vi "Calculate_Cost_F()-4.vi"(0 "[IN] Subtracks":T2(array[cluster]), 1 "[IN] Still connected\ntracks in group":T1, 2 "[IN] Max angle":dbl, 3 "[IN] Areas particles\nPrimary Detected":dbl[][](array[numeric]), 7 "[IN] Index of Earliest \nProblem Point Inside":i32, 9 "[IN] # of Longest track\nInside the Tracks Group":i32, 11 "error IN":errorcluster, 12 "[IN] Primary \n(X,Y) Detected":dbl[][](array[numeric]), 13 "[IN] Potentially\nMoving (X,Y)":dbl[][](array[numeric]), 14 "[IN] Dot matrix with statuses \nfor potentially moving dots":i16[][](array[numeric])) -> (4 "[OUT] Cost function":i8[](array[numeric]), 15 "error OUT":errorcluster)   [LabVIEW 2013]
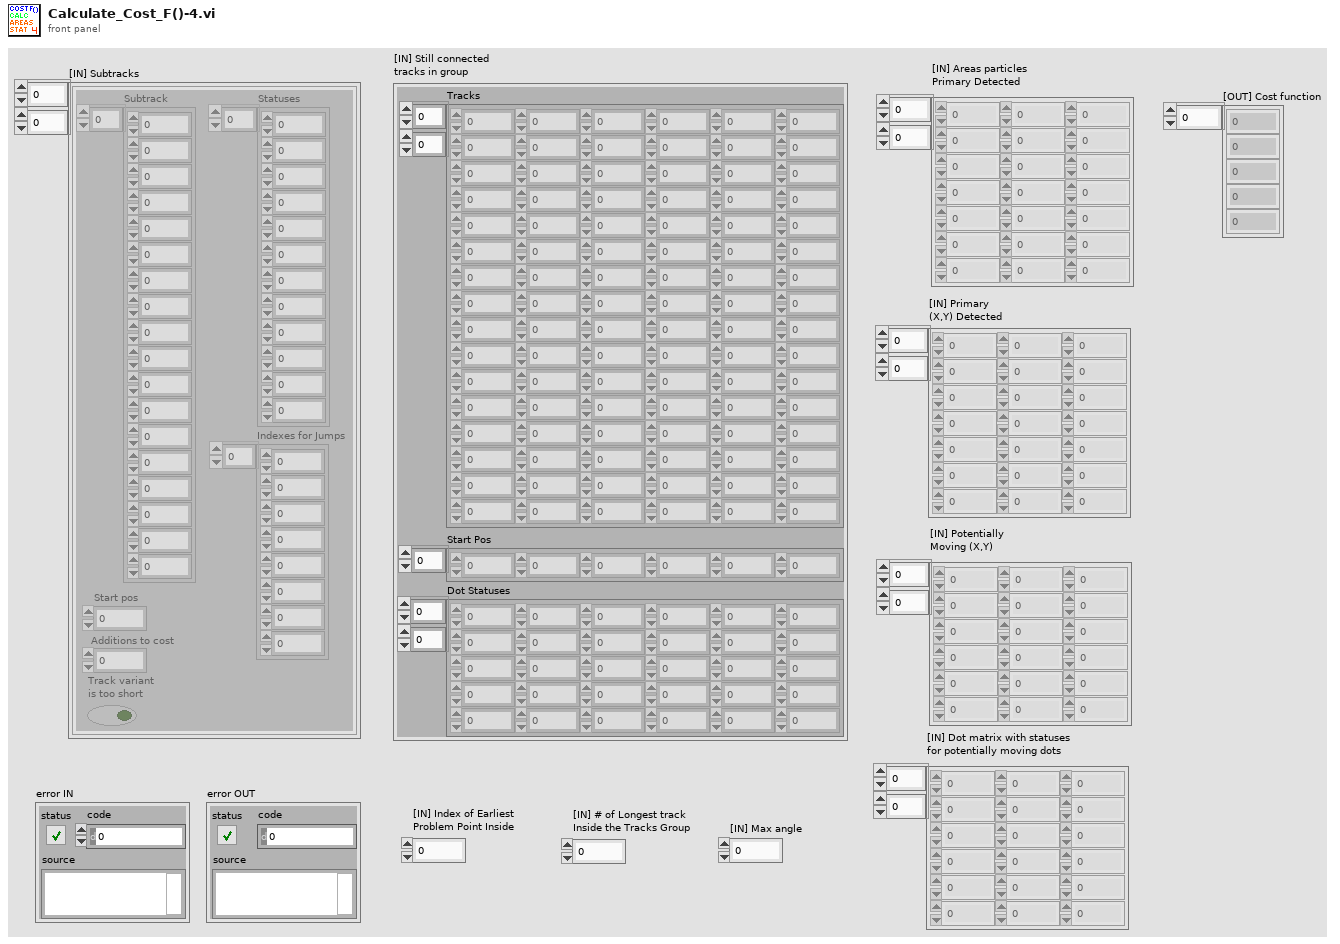
[diagram p1: front panel]
types:
  T1 = cluster{"Tracks":dbl[][], "Start Pos":i32[], "Dot Statuses":i16[][]}
  T2 = cluster{"Subtrack":dbl[], "Statuses":i16[], "Start pos":i32, "Additions to cost":i32, "Track variant \nis too short":bool, "Indexes for Jumps":i32[]}[][]
  T3 = cluster{"Subtrack":dbl[], "Statuses":i16[], "Start pos":i32, "Additions to cost":i32, "Track variant \nis too short":bool, "Indexes for Jumps":i32[]}[]
  T4 = cluster{"Subtrack":dbl[], "Statuses":i16[], "Start pos":i32, "Additions to cost":i32, "Track variant \nis too short":bool, "Indexes for Jumps":i32[]}
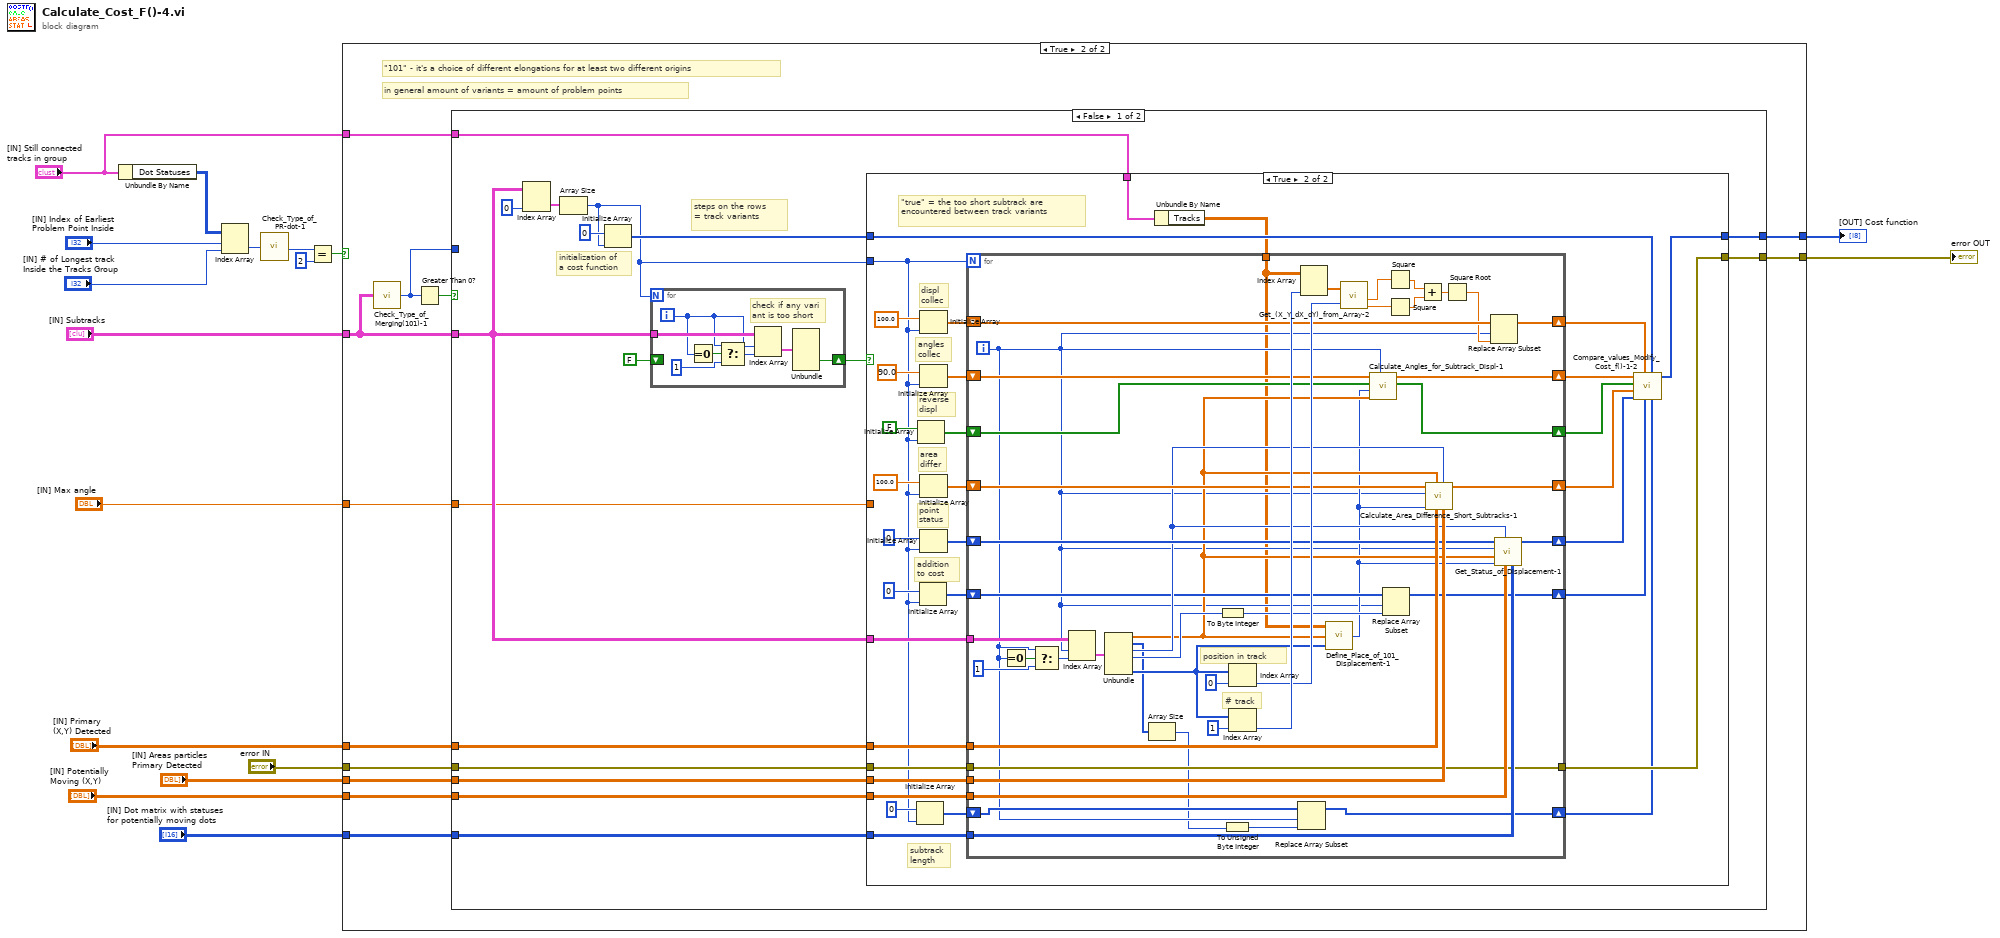
[diagram p0: block diagram]
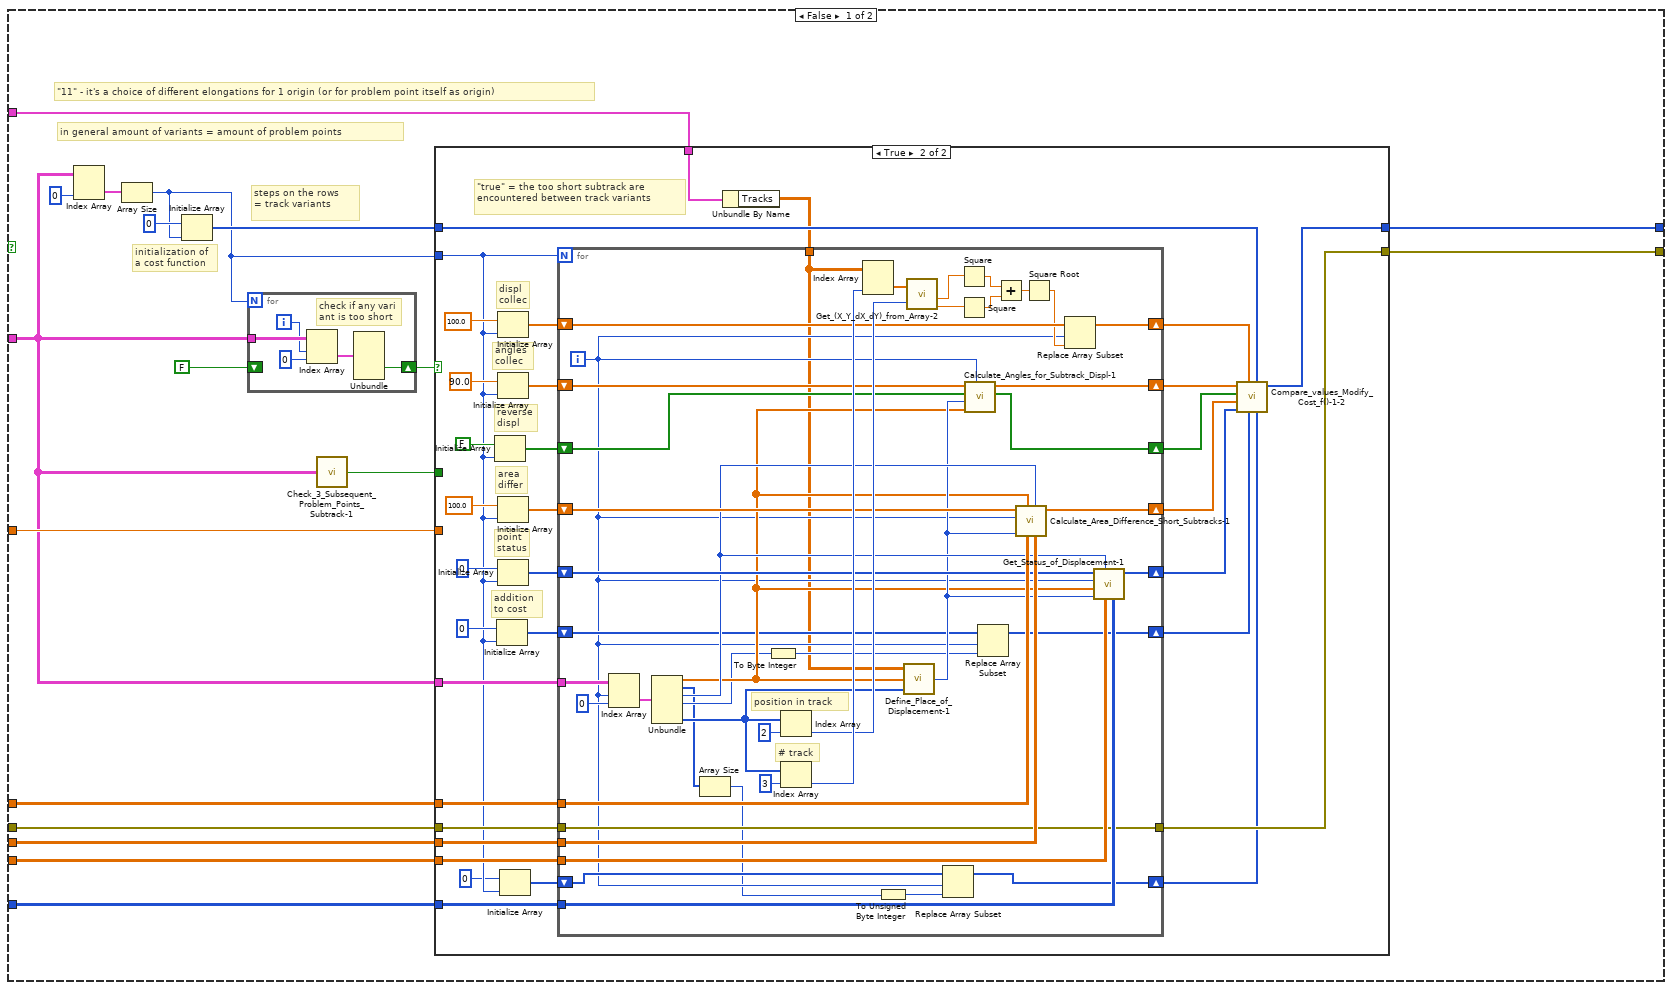
[diagram p2: hidden frame]
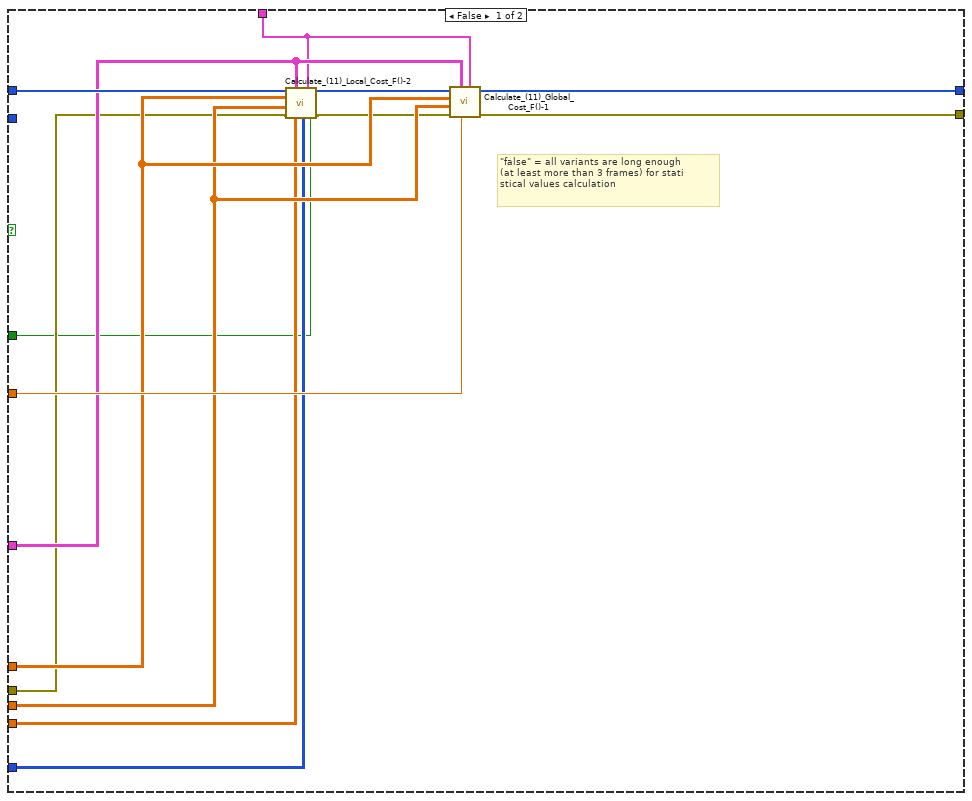
[diagram p3: hidden frame]
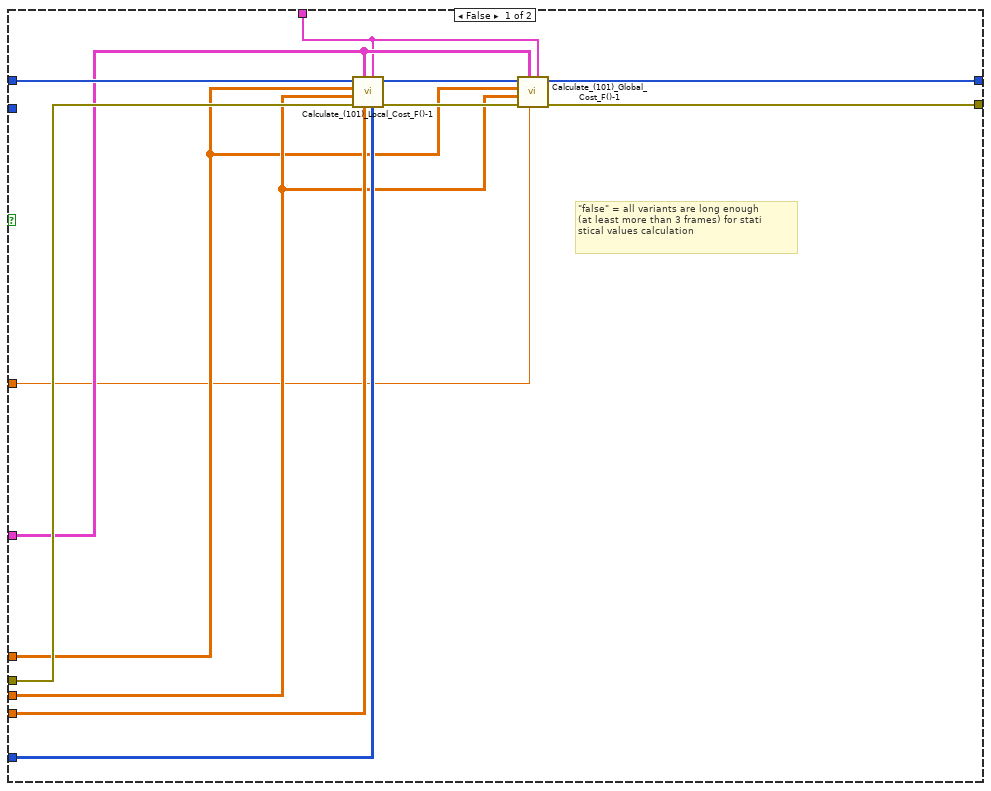
[diagram p4: hidden frame]
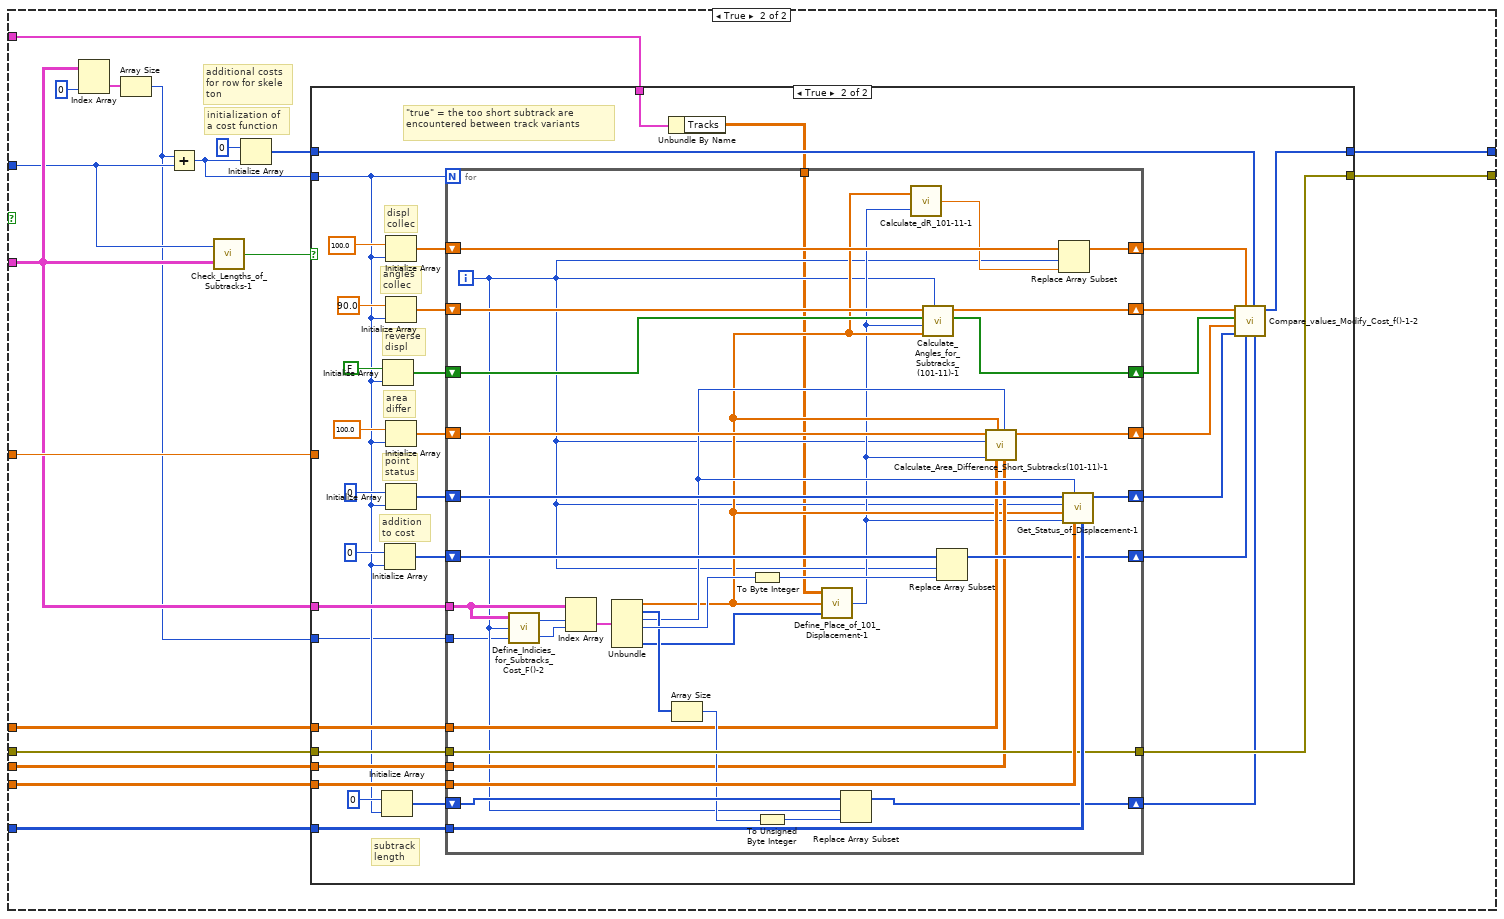
[diagram p5: hidden frame]
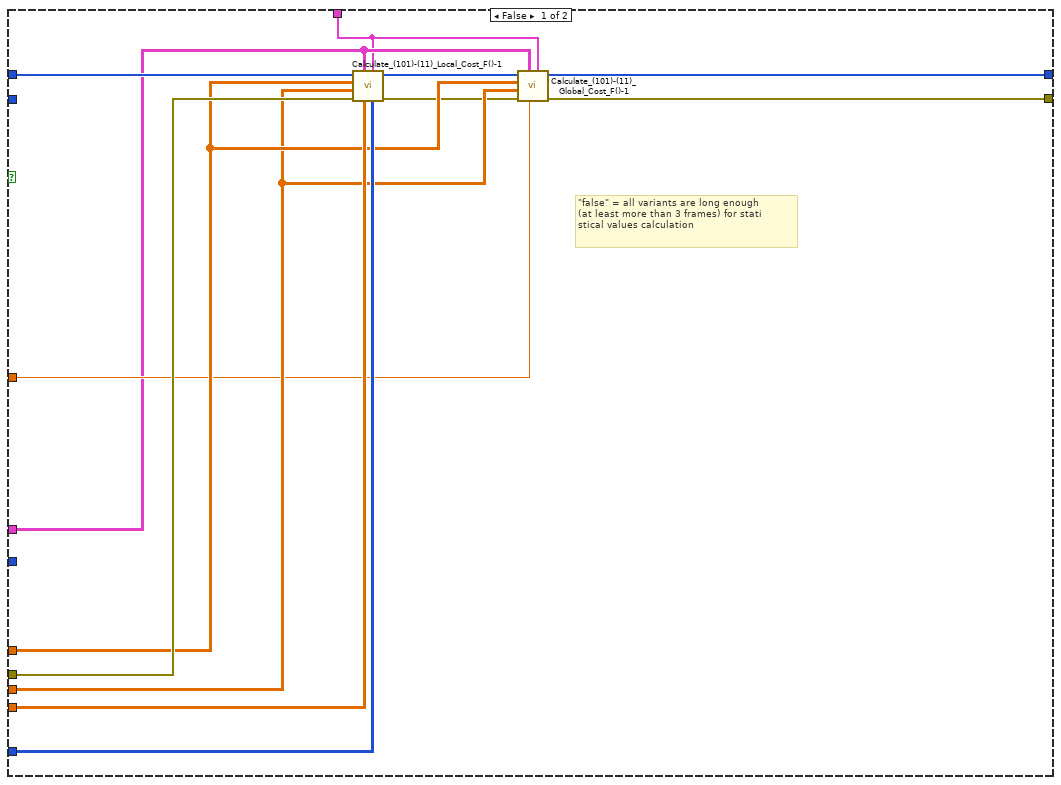
[diagram p6: hidden frame]
diagram:
  n1 = Unbundle By Name("[IN] Still connected\ntracks in group") -> ("Dot Statuses"=w15:i16[][])
  n2 = Index Array(array=w15, index (row)="[IN] Index of Earliest \nProblem Point Inside", index (col)="[IN] # of Longest track\nInside the Tracks Group") -> (element=w14:i16)
  n3 = call "Check_Type_of_PR-dot-1.vi"("[IN] dot status"=w14) -> ("[OUT] Type of\nproblem dot"=w17:i32)
  n4 = Equal?(x=w17, y=2) -> (x = y?=w13:bool)
  n5 = case shown="True" w13 {
    tunnel: "[IN] Subtracks" -> [w19 w135]
    tunnel: "[IN] Still connected\ntracks in group" -> [w29 w132]
    tunnel: "[IN] Primary \n(X,Y) Detected" -> [w28 w142]
    tunnel: "[IN] Areas particles\nPrimary Detected" -> [w27 w140]
    tunnel: "[IN] Potentially\nMoving (X,Y)" -> [w26 w139]
    tunnel: "[IN] Dot matrix with statuses \nfor potentially moving dots" -> [w25 w138]
    tunnel: "error IN" -> [w24 w141]
    tunnel: "[IN] Max angle" -> [w23 w143]
    tunnel: [w22 w137] -> w2
    tunnel: [w21 w136] -> w1
    frame False {
      # "initialization of \na cost function"
      # "steps on the rows\n= track variants"
      # "in general amount of variants = amount of problem points"
      # "\"11\" - it's a choice of different elongations for 1 origin (or for problem point itself as origin)"
      n6 = Index Array(array=w19, index (col)=0 ("disabled index (col)")) -> (element=w34:T3)  [unwired: 1 in]
      n7 = Array Size(array=w34) -> (size(s)=w20:i32)
      n8 = Initialize Array(i8 0, w20) -> (w30:i8[])
      n9 = for {
        N: w20 -> [_]
        tunnel: w19 -> [w131]
        shift-right: [w127] -> w31
        shift-left: FALSE -> [_]
        i -> [w128]
        # "check if any vari\nant is too short"
        n10 = Index Array(array=w131, index (row)=w128, index (col)=0 ("disabled index (col)")) -> (element=w129:T4)
        n11 = Unbundle(w129) -> ("Track variant \nis too short"=w127:bool)  [unwired: 5 out]
      }
      n12 = call "Check_3_Subsequent_Problem_Points_Subtrack-1.vi"("[IN] Subtracks"=w19) -> ("[OUT] 3 Subsequent problem points in subtrack"=w18:bool)
      n13 = case shown="True" w31 {
        tunnel: w30 -> [w46 w58]
        tunnel: w20 -> [_ w63]
        tunnel: w19 -> [w45 w82]
        tunnel: w29 -> [w44 w51]
        tunnel: w28 -> [w43 w73]
        tunnel: w27 -> [w42 w72]
        tunnel: w26 -> [w40 w69]
        tunnel: w25 -> [w39 w68]
        tunnel: w24 -> [w41 w65]
        tunnel: w23 -> [w49 _]
        tunnel: [w48 w57] -> w22
        tunnel: [w47 w64] -> w21
        tunnel: w18 -> [w36 _]
        frame False {
          # "\"false\" = all variants are long enough\n(at least more than 3 frames) for stati\nstical values calculation"
          n14 = call "Calculate_(11)_Local_Cost_F()-2.vi"("[IN] Cost function"=w46, "[IN] Subtracks"=w45, "[IN] Still connected\ntracks in group"=w44, "[IN] Primary \n(X,Y) Detected"=w43, "[IN] Areas particles\nPrimary Detected"=w42, "error IN"=w41, "[IN] Potentially\nMoving (X,Y)"=w40, "[IN] Dot matrix with statuses \nfor potentially moving dots"=w39, "[IN] 3 Subsequent problem points in subtrack"=w36) -> ("[OUT] Cost function"=w37:i8[], "error OUT"=w38:errorcluster)  [unwired: 5 in]
          n15 = call "Calculate_(11)_Global_Cost_F()-1.vi"("[IN] Still connect\ned tracks in group"=w44, "[IN] Max angle"=w49, "[IN] Subtracks"=w45, "error IN"=w38, "[IN] Areas particles\nPrimary Detected"=w42, "[IN] Primary \n(X,Y) Detected"=w43, "[IN] Cost function"=w37) -> ("error OUT"=w47:errorcluster, "[OUT] Cost function"=w48:i8[])  [unwired: 3 in]
        }
        frame True {
          # "addition \nto cost"
          # "point\nstatus"
          # "area \ndiffer"
          # "reverse \ndispl"
          # "angles \ncollec"
          # "displ \ncollec"
          # "\"true\" = the too short subtrack are \nencountered between track variants"
          n16 = Initialize Array(FALSE, w63) -> (w76:bool[])
          n17 = Initialize Array(i8 0, w63) -> (w66:i8[])
          n18 = Initialize Array(100.0, w63) -> (w80:dbl[])
          n19 = Initialize Array(90.0, w63) -> (w78:dbl[])
          n20 = Initialize Array(100.0, w63) -> (w74:dbl[])
          n21 = Initialize Array(i16 0, w63) -> (w70:i16[])
          n22 = Initialize Array(u8 0, w63) -> (w61:u8[])
          n23 = Unbundle By Name(w51) -> ("Tracks"=w50:dbl[][])
          n24 = for {
            N: w63 -> [_]
            tunnel: w82 -> [w126]
            shift-right: [w117] -> w59
            shift-left: w80 -> [w118]
            shift-right: [w114] -> w60
            shift-left: w78 -> [w115]
            shift-right: [w112] -> w56
            shift-left: w76 -> [w113]
            tunnel: w73 -> [w108]
            tunnel: w72 -> [w110]
            shift-right: [w109] -> w55
            shift-left: w74 -> [w111]
            tunnel: w69 -> [w103]
            tunnel: w68 -> [w102]
            shift-right: [w101] -> w54
            shift-left: w70 -> [w107]
            shift-right: [w97] -> w53
            shift-left: w66 -> [w100]
            tunnel: w65 -> [w90]
            tunnel: [w90] -> w64
            shift-right: [w87] -> w52
            shift-left: w61 -> [w88]
            tunnel: w50 -> [w83]
            i -> [w86]
            # "# track"
            # "position in track"
            n25 = Index Array(array=w126, index (row)=w86, index (col)=0 ("disabled index (col)")) -> (element=w124:T4)
            n26 = Unbundle(w124) -> ("Subtrack"=w104:dbl[], "Statuses"=w89:i16[], "Start pos"=w106:i32, "Additions to cost"=w99:i32, "Indexes for Jumps"=w116:i32[])  [unwired: 1 out]
            n27 = Array Size(array=w89) -> (size(s)=w85:i32)
            n28 = To Byte Integer(number=w99) -> (8bit integer=w98:i8)
            n29 = Index Array(array=w116, index=2) -> (element=w119:i32)
            n30 = Index Array(array=w116, index=3) -> (element=w121:i32)
            n31 = Index Array(array=w83, index (col)=w121) -> (element=w120:dbl[])  [unwired: 1 in]
            n32 = To Unsigned Byte Integer(number=w85) -> (unsigned 8bit integer=w84:u8)
            n33 = call "Define_Place_of_Displacement-1.vi"("[IN] Indexes for Jumps"=w116, "[IN] Subtrack"=w104, "[IN] Tracks"=w83) -> ("[OUT] Index of \"11\" Dis\nplacement in Subtrack"=w105:i32)  [unwired: 2 in]
            n34 = call "Get_(X_Y_dX_dY)_from_Array-2.vi"("(X,Y,dX,dY)"=w120, "Index of Displacement"=w119) -> ("dX"=w93:dbl, "dY"=w92:dbl)  [unwired: 2 out]
            n35 = Replace Array Subset(array=w88, new element=w84, index=w86) -> (w87:u8[])
            n36 = Square(x=w93) -> (x^2=w96:dbl)
            n37 = Square(x=w92) -> (x^2=w95:dbl)
            n38 = call "Calculate_Angles_for_Subtrack_Displ-1.vi"("[IN] Index of subtrack"=w86, "[IN] Subtrack"=w104, "[IN] Index of \"11\" Dis-\nplacement in Subtrack"=w105, "[IN] Reverse Displ or Not"=w113, "[IN] Array with Angles \nBetween Displacement"=w115) -> ("[OUT] Reverse displacement or not"=w112:bool[], "[OUT] Angles betwe\nen two displacements"=w114:dbl[])  [unwired: 3 in]
            n39 = Replace Array Subset(array=w100, new element=w98, index=w86) -> (w97:i8[])
            n40 = Add(x=w96, y=w95) -> (x+y=w94:dbl)
            n41 = call "Calculate_Area_Difference_Short_Subtracks-1.vi"("[IN] Areas particles\nPrimary Detected"=w110, "[IN] Start pos"=w106, "[IN] Primary \n(X,Y) Detected"=w108, "[IN] Subtrack"=w104, "[IN] Index of \"11\" Dis-\nplacement in Subtrack"=w105, "[IN] Index of\n subtrack"=w86, "[IN] Areas \ndifference"=w111) -> ("[OUT] Areas \ndifference"=w109:dbl[])  [unwired: 4 in]
            n42 = Square Root(x=w94) -> (sqrt(x)=w91:dbl)
            n43 = Replace Array Subset(array=w118, new element=w91, index=w86) -> (w117:dbl[])
            n44 = call "Get_Status_of_Displacement-1.vi"("[IN] Dot matrix with statuses\nfor potentially moving dots"=w102, "[IN] Potentially\nMoving (X,Y)"=w103, "[IN] Start pos"=w106, "[IN] Index of Problem\nPoint in Subtrack"=w105, "[IN] Subtrack"=w104, "[IN] Index of\n subtrack"=w86, "[IN] Displace-\nment Statuses"=w107) -> ("[OUT] Displace\nment Statuses"=w101:i16[])  [unwired: 4 in]
          }
          n45 = call "Compare_values_Modify_Cost_f()-1-2.vi"("[IN] Track Length"=w52, "[IN] Cost function"=w58, "[IN] Additions to cost"=w53, "[IN] Array of displa\ncement differences"=w59, "[IN] Statuses of points"=w54, "[IN] Areas \ndifferences"=w55, "[IN] Reverse or not"=w56, "[IN] Angles betwe\nen displacements"=w60) -> ("[OUT] Cost function"=w57:i8[])  [unwired: 3 in]
        }
      }
    }
    frame True {
      # "in general amount of variants = amount of problem points"
      # "\"101\" - it's a choice of different elongations for at least two different origins"
      n46 = call "Check_Type_of_Merging(101)-1.vi"("[IN] Subtracks"=w135) -> ("[OUT] # of Additional Costs"=w133:i32)
      n47 = Greater Than 0?(x=w133) -> (x > 0?=w134:bool)
      n48 = case shown="False" w134 {
        tunnel: w132 -> [w153 w267]
        tunnel: w135 -> [w152 w266]
        tunnel: w143 -> [w151 w268]
        tunnel: w142 -> [w150 w273]
        tunnel: w141 -> [w149 w272]
        tunnel: w140 -> [w148 w271]
        tunnel: w139 -> [w147 w270]
        tunnel: w138 -> [w146 w269]
        tunnel: [w145 w261] -> w137
        tunnel: [w144 w260] -> w136
        tunnel: w133 -> [_ w263]
        frame False {
          # "initialization of \na cost function"
          # "steps on the rows\n= track variants"
          n49 = Index Array(array=w152, index (col)=0 ("disabled index (col)")) -> (element=w159:T3)  [unwired: 1 in]
          n50 = Array Size(array=w159) -> (size(s)=w154:i32)
          n51 = Initialize Array(i8 0, w154) -> (w155:i8[])
          n52 = for {
            N: w154 -> [_]
            tunnel: w152 -> [w259]
            shift-right: [w257] -> w156
            shift-left: FALSE -> [_]
            i -> [w253]
            # "check if any vari\nant is too short"
            n53 = Equal To 0?(x=w253) -> (x = 0?=w256:bool)
            n54 = Select(t=w253, s=w256, f=1) -> (s? t:f=w254:i32)
            n55 = Index Array(array=w259, index (row)=w253, index (col)=w254) -> (element=w258:T4)
            n56 = Unbundle(w258) -> ("Track variant \nis too short"=w257:bool)  [unwired: 5 out]
          }
          n57 = case shown="True" w156 {
            tunnel: w155 -> [w173 w182]
            tunnel: w154 -> [_ w186]
            tunnel: w152 -> [w165 w206]
            tunnel: w153 -> [w164 w175]
            tunnel: w150 -> [w167 w197]
            tunnel: w148 -> [w168 w196]
            tunnel: w147 -> [w172 w193]
            tunnel: w146 -> [w170 w192]
            tunnel: w149 -> [w171 w189]
            tunnel: w151 -> [w163 _]
            tunnel: [w162 w181] -> w145
            tunnel: [w161 w188] -> w144
            frame False {
              # "\"false\" = all variants are long enough\n(at least more than 3 frames) for stati\nstical values calculation"
              n58 = call "Calculate_(101)_Local_Cost_F()-1.vi"("[IN] Dot matrix with statuses \nfor potentially moving dots"=w170, "[IN] Still connected\ntracks in group"=w164, "[IN] Potentially\nMoving (X,Y)"=w172, "[IN] Subtracks"=w165, "error IN"=w171, "[IN] Areas particles\nPrimary Detected"=w168, "[IN] Primary \n(X,Y) Detected"=w167, "[IN] Cost function"=w173) -> ("error OUT"=w169:errorcluster, "[OUT] Cost function"=w166:i8[])  [unwired: 2 in]
              n59 = call "Calculate_(101)_Global_Cost_F()-1.vi"("[IN] Still connect\ned tracks in group"=w164, "[IN] Max angle"=w163, "[IN] Subtracks"=w165, "error IN"=w169, "[IN] Areas particles\nPrimary Detected"=w168, "[IN] Primary \n(X,Y) Detected"=w167, "[IN] Cost function"=w166) -> ("error OUT"=w161:errorcluster, "[OUT] Cost function"=w162:i8[])  [unwired: 3 in]
            }
            frame True {
              # "subtrack\nlength"
              # "addition \nto cost"
              # "point\nstatus"
              # "area \ndiffer"
              # "reverse \ndispl"
              # "angles \ncollec"
              # "displ \ncollec"
              # "\"true\" = the too short subtrack are \nencountered between track variants"
              n60 = Initialize Array(u8 0, w186) -> (w185:u8[])
              n61 = Initialize Array(FALSE, w186) -> (w200:bool[])
              n62 = Initialize Array(i8 0, w186) -> (w190:i8[])
              n63 = Initialize Array(100.0, w186) -> (w204:dbl[])
              n64 = Initialize Array(90.0, w186) -> (w202:dbl[])
              n65 = Initialize Array(100.0, w186) -> (w198:dbl[])
              n66 = Initialize Array(i16 0, w186) -> (w194:i16[])
              n67 = Unbundle By Name(w175) -> ("Tracks"=w174:dbl[][])
              n68 = for {
                N: w186 -> [_]
                tunnel: w206 -> [w252]
                shift-right: [w244] -> w183
                shift-left: w204 -> [w245]
                shift-right: [w242] -> w184
                shift-left: w202 -> [w243]
                shift-right: [w240] -> w177
                shift-left: w200 -> [w241]
                tunnel: w197 -> [w236]
                tunnel: w196 -> [w238]
                shift-right: [w237] -> w178
                shift-left: w198 -> [w239]
                tunnel: w193 -> [w233]
                tunnel: w192 -> [w232]
                shift-right: [w231] -> w179
                shift-left: w194 -> [w235]
                shift-right: [w227] -> w180
                shift-left: w190 -> [w230]
                tunnel: w189 -> [w220]
                tunnel: [w220] -> w188
                shift-right: [w210] -> w176
                shift-left: w185 -> [w212]
                tunnel: w174 -> [w207]
                i -> [w211]
                # "# track"
                # "position in track"
                n69 = Equal To 0?(x=w211) -> (x = 0?=w219:bool)
                n70 = Select(t=w211, s=w219, f=1) -> (s? t:f=w217:i32)
                n71 = Index Array(array=w252, index (row)=w211, index (col)=w217) -> (element=w251:T4)
                n72 = Unbundle(w251) -> ("Subtrack"=w216:dbl[], "Statuses"=w213:i16[], "Start pos"=w234:i32, "Additions to cost"=w229:i32, "Indexes for Jumps"=w215:i32[])  [unwired: 1 out]
                n73 = Array Size(array=w213) -> (size(s)=w209:i32)
                n74 = To Byte Integer(number=w229) -> (8bit integer=w228:i8)
                n75 = To Unsigned Byte Integer(number=w209) -> (unsigned 8bit integer=w208:u8)
                n76 = Index Array(array=w215, index=0) -> (element=w246:i32)
                n77 = Index Array(array=w215, index=1) -> (element=w248:i32)
                n78 = Replace Array Subset(array=w212, new element=w208, index=w211) -> (w210:u8[])
                n79 = Index Array(array=w207, index (col)=w248) -> (element=w247:dbl[])  [unwired: 1 in]
                n80 = call "Define_Place_of_101_Displacement-1.vi"("[IN] Indexes for Jumps"=w215, "[IN] Subtrack"=w216, "[IN] Tracks"=w207) -> ("[OUT] Index of \"11\" Dis\nplacement in Subtrack"=w214:i32)  [unwired: 2 in]
                n81 = call "Get_(X_Y_dX_dY)_from_Array-2.vi"("(X,Y,dX,dY)"=w247, "Index of Displacement"=w246) -> ("dX"=w223:dbl, "dY"=w222:dbl)  [unwired: 2 out]
                n82 = call "Calculate_Angles_for_Subtrack_Displ-1.vi"("[IN] Index of subtrack"=w211, "[IN] Subtrack"=w216, "[IN] Index of \"11\" Dis-\nplacement in Subtrack"=w214, "[IN] Reverse Displ or Not"=w241, "[IN] Array with Angles \nBetween Displacement"=w243) -> ("[OUT] Reverse displacement or not"=w240:bool[], "[OUT] Angles betwe\nen two displacements"=w242:dbl[])  [unwired: 3 in]
                n83 = Replace Array Subset(array=w230, new element=w228, index=w211) -> (w227:i8[])
                n84 = Square(x=w223) -> (x^2=w226:dbl)
                n85 = Square(x=w222) -> (x^2=w225:dbl)
                n86 = Add(x=w226, y=w225) -> (x+y=w224:dbl)
                n87 = call "Calculate_Area_Difference_Short_Subtracks-1.vi"("[IN] Areas particles\nPrimary Detected"=w238, "[IN] Start pos"=w234, "[IN] Primary \n(X,Y) Detected"=w236, "[IN] Subtrack"=w216, "[IN] Index of \"11\" Dis-\nplacement in Subtrack"=w214, "[IN] Index of\n subtrack"=w211, "[IN] Areas \ndifference"=w239) -> ("[OUT] Areas \ndifference"=w237:dbl[])  [unwired: 4 in]
                n88 = Square Root(x=w224) -> (sqrt(x)=w221:dbl)
                n89 = Replace Array Subset(array=w245, new element=w221, index=w211) -> (w244:dbl[])
                n90 = call "Get_Status_of_Displacement-1.vi"("[IN] Dot matrix with statuses\nfor potentially moving dots"=w232, "[IN] Potentially\nMoving (X,Y)"=w233, "[IN] Start pos"=w234, "[IN] Index of Problem\nPoint in Subtrack"=w214, "[IN] Subtrack"=w216, "[IN] Index of\n subtrack"=w211, "[IN] Displace-\nment Statuses"=w235) -> ("[OUT] Displace\nment Statuses"=w231:i16[])  [unwired: 4 in]
              }
              n91 = call "Compare_values_Modify_Cost_f()-1-2.vi"("[IN] Track Length"=w176, "[IN] Cost function"=w182, "[IN] Additions to cost"=w180, "[IN] Array of displa\ncement differences"=w183, "[IN] Statuses of points"=w179, "[IN] Areas \ndifferences"=w178, "[IN] Reverse or not"=w177, "[IN] Angles betwe\nen displacements"=w184) -> ("[OUT] Cost function"=w181:i8[])  [unwired: 3 in]
            }
          }
        }
        frame True {
          # "additional costs\nfor row for skele\nton"
          # "initialization of \na cost function"
          n92 = Index Array(array=w266, index (col)=0 ("disabled index (col)")) -> (element=w276:T3)  [unwired: 1 in]
          n93 = Array Size(array=w276) -> (size(s)=w262:i32)
          n94 = Add(x=w262, y=w263) -> (x+y=w264:i32)
          n95 = call "Check_Lengths_of_Subtracks-1.vi"("[IN] Subtracks"=w266, "[IN] Number of Additi\nonal Costs (Subtracks)"=w263) -> ("[OUT[ Is between subtracks\npresented too short one?"=w265:bool)
          n96 = Initialize Array(i8 0, w264) -> (w274:i8[])
          n97 = case shown="True" w265 {
            tunnel: w274 -> [w289 w300]
            tunnel: w264 -> [_ w304]
            tunnel: w266 -> [w281 w324]
            tunnel: w267 -> [w280 w292]
            tunnel: w273 -> [w285 w315]
            tunnel: w271 -> [w284 w314]
            tunnel: w270 -> [w288 w311]
            tunnel: w269 -> [w287 w310]
            tunnel: w272 -> [w290 w307]
            tunnel: w268 -> [w282 _]
            tunnel: [w279 w299] -> w261
            tunnel: [w278 w306] -> w260
            tunnel: w262 -> [_ w293]
            frame False {
              # "\"false\" = all variants are long enough\n(at least more than 3 frames) for stati\nstical values calculation"
              n98 = call "Calculate_(101)-(11)_Local_Cost_F()-1.vi"("[IN] Dot matrix with statuses \nfor potentially moving dots"=w287, "[IN] Still connected\ntracks in group"=w280, "[IN] Potentially\nMoving (X,Y)"=w288, "[IN] Subtracks"=w281, "error IN"=w290, "[IN] Areas particles\nPrimary Detected"=w284, "[IN] Primary \n(X,Y) Detected"=w285, "[IN] Cost function"=w289) -> ("error OUT"=w283:errorcluster, "[OUT] Cost function"=w286:i8[])  [unwired: 2 in]
              n99 = call "Calculate_(101)-(11)_Global_Cost_F()-1.vi"("[IN] Still connect\ned tracks in group"=w280, "[IN] Max angle"=w282, "[IN] Subtracks"=w281, "error IN"=w283, "[IN] Areas particles\nPrimary Detected"=w284, "[IN] Primary \n(X,Y) Detected"=w285, "[IN] Cost function"=w286) -> ("error OUT"=w278:errorcluster, "[OUT] Cost function"=w279:i8[])  [unwired: 3 in]
            }
            frame True {
              # "subtrack\nlength"
              # "addition \nto cost"
              # "point\nstatus"
              # "area \ndiffer"
              # "reverse \ndispl"
              # "angles \ncollec"
              # "displ \ncollec"
              # "\"true\" = the too short subtrack are \nencountered between track variants"
              n100 = Initialize Array(u8 0, w304) -> (w303:u8[])
              n101 = Initialize Array(FALSE, w304) -> (w318:bool[])
              n102 = Initialize Array(i8 0, w304) -> (w308:i8[])
              n103 = Initialize Array(100.0, w304) -> (w322:dbl[])
              n104 = Initialize Array(90.0, w304) -> (w320:dbl[])
              n105 = Initialize Array(100.0, w304) -> (w316:dbl[])
              n106 = Initialize Array(i16 0, w304) -> (w312:i16[])
              n107 = Unbundle By Name(w292) -> ("Tracks"=w291:dbl[][])
              n108 = for {
                N: w304 -> [_]
                tunnel: w324 -> [w330]
                shift-right: [w358] -> w301
                shift-left: w322 -> [w359]
                shift-right: [w338] -> w302
                shift-left: w320 -> [w341]
                shift-right: [w339] -> w295
                shift-left: w318 -> [w340]
                tunnel: w315 -> [w333]
                tunnel: w314 -> [w334]
                shift-right: [w335] -> w296
                shift-left: w316 -> [w337]
                tunnel: w311 -> [w356]
                tunnel: w310 -> [w355]
                shift-right: [w354] -> w297
                shift-left: w312 -> [w357]
                shift-right: [w350] -> w298
                shift-left: w308 -> [w353]
                tunnel: w307 -> [w349]
                tunnel: [w349] -> w306
                shift-right: [w347] -> w294
                shift-left: w303 -> [w348]
                tunnel: w293 -> [w326]
                tunnel: w291 -> [w325]
                i -> [w327]
                n109 = call "Define_Indicies_for_Subtracks_Cost_F()-2.vi"("[IN] Number of Rows"=w326, "[IN] Current index"=w327, "[IN] Subtracks"=w330) -> ("[OUT] Column \n# for Subtrack"=w328:i32, "[OUT] Row # \nfor Subtrack"=w329:i32)
                n110 = Index Array(array=w330, index (row)=w329, index (col)=w328) -> (element=w360:T4)
                n111 = Unbundle(w360) -> ("Subtrack"=w332:dbl[], "Statuses"=w344:i16[], "Start pos"=w336:i32, "Additions to cost"=w352:i32, "Indexes for Jumps"=w343:i32[])  [unwired: 1 out]
                n112 = Array Size(array=w344) -> (size(s)=w346:i32)
                n113 = To Byte Integer(number=w352) -> (8bit integer=w351:i8)
                n114 = To Unsigned Byte Integer(number=w346) -> (unsigned 8bit integer=w345:u8)
                n115 = call "Define_Place_of_101_Displacement-1.vi"("[IN] Indexes for Jumps"=w343, "[IN] Subtrack"=w332, "[IN] Tracks"=w325) -> ("[OUT] Index of \"11\" Dis\nplacement in Subtrack"=w331:i32)  [unwired: 2 in]
                n116 = Replace Array Subset(array=w348, new element=w345, index=w327) -> (w347:u8[])
                n117 = call "Calculate_dR_101-11-1.vi"("[IN] Index of \"101\"\nDisplacement"=w331, "[IN] Subtrack"=w332) -> ("[OUT] Displacement average"=w342:dbl)
                n118 = call "Calculate_Angles_for_Subtracks_(101-11)-1.vi"("[IN] Index of subtrack"=w327, "[IN] Subtrack"=w332, "[IN] Index of \"101\" Dis-\nplacement in Subtrack"=w331, "[IN] Reverse Displ or Not"=w340, "[IN] Array with Angles \nBetween Displacement"=w341) -> ("[OUT] Reverse displacement or not"=w339:bool[], "[OUT] Angles betwe\nen two displacements"=w338:dbl[])  [unwired: 3 in]
                n119 = Replace Array Subset(array=w353, new element=w351, index=w327) -> (w350:i8[])
                n120 = call "Calculate_Area_Difference_Short_Subtracks(101-11)-1.vi"("[IN] Areas particles\nPrimary Detected"=w334, "[IN] Start pos"=w336, "[IN] Primary \n(X,Y) Detected"=w333, "[IN] Subtrack"=w332, "[IN] Index of \"101\" Dis-\nplacement in Subtrack"=w331, "[IN] Index of\n subtrack"=w327, "[IN] Areas \ndifference"=w337) -> ("[OUT] Areas differen\nce (101 + 11 points)"=w335:dbl[])  [unwired: 4 in]
                n121 = Replace Array Subset(array=w359, new element=w342, index=w327) -> (w358:dbl[])
                n122 = call "Get_Status_of_Displacement-1.vi"("[IN] Dot matrix with statuses\nfor potentially moving dots"=w355, "[IN] Potentially\nMoving (X,Y)"=w356, "[IN] Start pos"=w336, "[IN] Index of Problem\nPoint in Subtrack"=w331, "[IN] Subtrack"=w332, "[IN] Index of\n subtrack"=w327, "[IN] Displace-\nment Statuses"=w357) -> ("[OUT] Displace\nment Statuses"=w354:i16[])  [unwired: 4 in]
              }
              n123 = call "Compare_values_Modify_Cost_f()-1-2.vi"("[IN] Track Length"=w294, "[IN] Cost function"=w300, "[IN] Additions to cost"=w298, "[IN] Array of displa\ncement differences"=w301, "[IN] Statuses of points"=w297, "[IN] Areas \ndifferences"=w296, "[IN] Reverse or not"=w295, "[IN] Angles betwe\nen displacements"=w302) -> ("[OUT] Cost function"=w299:i8[])  [unwired: 3 in]
            }
          }
        }
      }
    }
  }
  "error OUT" <- w1
  "[OUT] Cost function" <- w2
